vi "Read Leak State.vi"(8 "error in (no error)":errorcluster, 9 "timeout in ms (-1)":i32=-1, 10 "Leak Location":T1, 11 "Viewable Leak Queue In":refnum<queue>) -> (0 "error out":errorcluster, 1 "State Found?":bool, 2 "State Snapshot":T2, 3 "Viewable Leak Queue":refnum<queue>)   [LabVIEW 2017, in "LeakyViewable.lvlib" / "LeakyViewable.lvclass"]
uses:
  LeakyViewable.lvclass
  Leak Location.ctl
  Source/IViewable/IViewable/IViewable.lvclass
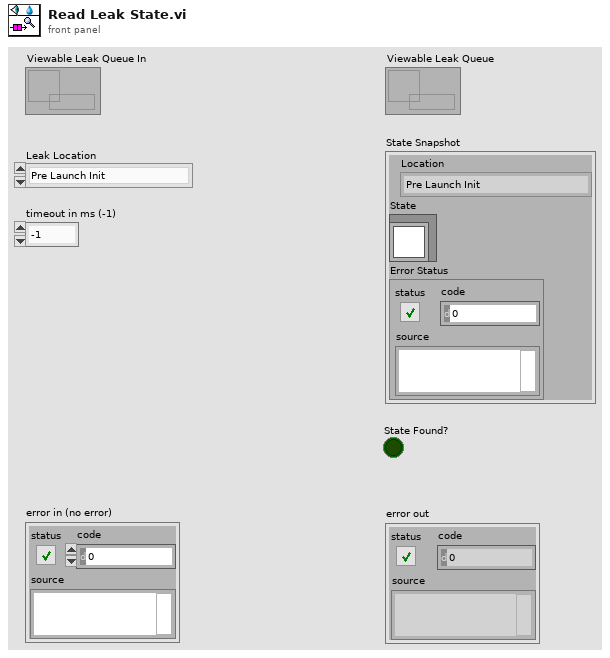
[diagram p1: front panel]
types:
  T1 = typedef "LeakyViewable.lvlib/LeakyViewable.lvclass/Leak Location.ctl" = enum16{"Pre Launch Init", "Entering Actor Core", "Actor Core", "Exiting Actor Core", "Stop Core", "Handle Error"}
  T2 = cluster{"Location":T1, "State":refnum<class "IViewable.lvclass">, "Error Status":errorcluster}
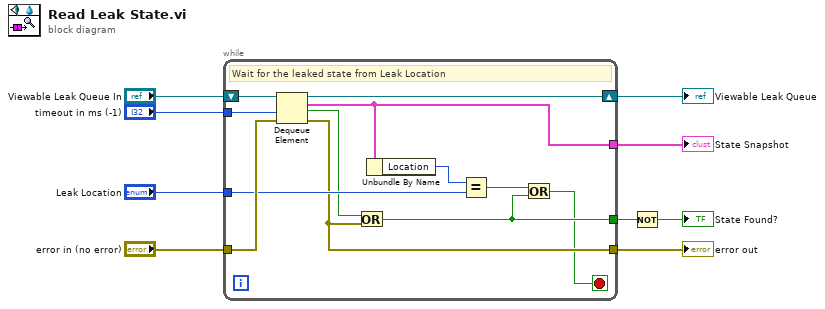
[diagram p0: block diagram]
diagram:
  n1 = while {
    tunnel: [w17] -> w3
    shift-right: [w21] -> w4
    shift-left: "Viewable Leak Queue In" -> [w20]
    tunnel: "timeout in ms (-1)" -> [w19]
    tunnel: [w13] -> w7
    tunnel: "error in (no error)" -> [w16]
    tunnel: "Leak Location" -> [w15]
    tunnel: [w11] -> w2
    stop <- w10 stop-if-true
    # "Wait for the leaked state from Leak Location"
    n2 = Dequeue Element(queue=w20, timeout in ms (-1)=w19, error in (no error)=w16) -> (queue out=w21:refnum<queue>, element=w17:T2, timed out?=w14:bool, error out=w13:errorcluster)
    n3 = Or(x=w14, y=w13) -> (x .or. y?=w11:bool)
    n4 = Unbundle By Name(w17) -> ("Location"=w18:T1)
    n5 = Equal?(x=w18, y=w15) -> (x = y?=w12:bool)
    n6 = Or(x=w12, y=w11) -> (x .or. y?=w10:bool)
  }
  "Viewable Leak Queue" <- w4
  "error out" <- w7
  "State Snapshot" <- w3
  n7 = Not(x=w2) -> (.not. x?=→"State Found?":bool)
